vi "ProbePlanSpreadsheet.vi"(0 "ProbePoints":T1(array[cluster])) -> (1 "Coordinates":string[][](table), 2 "Number of ProbePoints":i32)   [LabVIEW 2019]
doc: "Utility to fill a spreadsheet with probe region/point labels, coordinates, and whether they are enabled for movement with respect to the probe card."
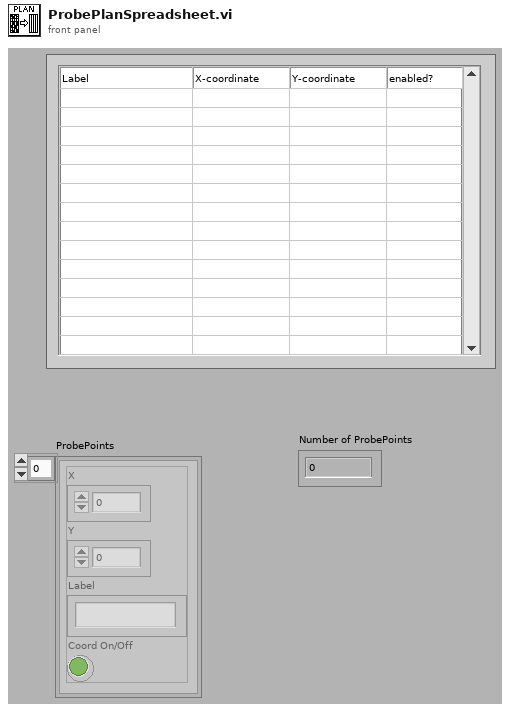
[diagram p1: front panel]
types:
  T1 = cluster{"X":dbl, "Y":dbl, "Label":string, "Coord On/Off":bool}[]
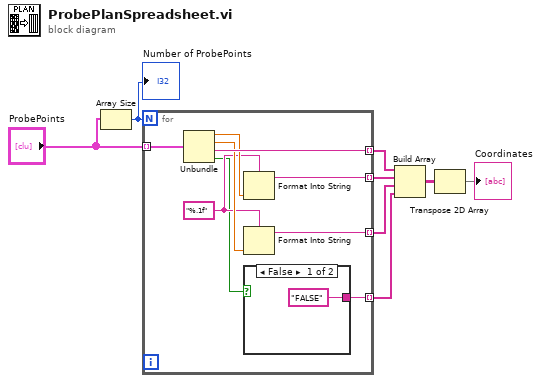
[diagram p0: block diagram]
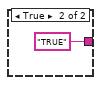
[diagram p2: hidden frame]
diagram:
  n1 = Array Size(array="ProbePoints") -> (size(s)=w8:i32)
  "Number of ProbePoints" <- w8
  n2 = for {
    N: w8 -> [_]
    tunnel: "ProbePoints" -> [w17] mode=indexing
    tunnel: [w16] -> w7 mode=indexing
    tunnel: [w14] -> w6 mode=indexing
    tunnel: [w11] -> w5 mode=indexing
    tunnel: [w9] -> w2 mode=indexing
    w12 = "%.1f" ("format string")
    n3 = Unbundle(w17) -> ("X"=w15:dbl, "Y"=w13:dbl, "Label"=w16:string, "Coord On/Off"=w10:bool)
    n4 = Format Into String(format string=w12, w15) -> (resulting string=w14:string)  [unwired: 2 in, 1 out]
    n5 = Format Into String(format string=w12, w13) -> (resulting string=w11:string)  [unwired: 2 in, 1 out]
    n6 = case shown="False" w10 {
      tunnel: ["FALSE" "TRUE"] -> w9
      frame False {
      }
      frame True {
      }
    }
  }
  n7 = Build Array(w7, w6, w5, w2) -> (w4:string[][])
  n8 = Transpose 2D Array(2D array=w4) -> (transposed array=→"Coordinates":string[][])
